vi "Dashboard Main.vi"() -> ()   [LabVIEW 2020]
uses:
  <vilib>/event_ctls.llb/eventvkey.ctl
  <vilib>/Rock Robotics/Network Tables/NT Read Numeric Array.vi
  <vilib>/Rock Robotics/WPI/Dashboard/WPI_DashboardLogging Global.vi
panel:
  in  "Camera Settings Right":T1={"Frame Rate"=30, "Compression"=30, "Size"=1, "DB Camera Config"=FALSE} {"Frame Rate" scale=1.0..30.0; "Compression" scale=100.0..-1.0; "Size" items=["640x480", "320x240", "160x120"]}
  in  "Camera Name Right":string(combo)="No Camera Selection"
  out "Camera Perf":string
  in  "Camera Settings":T1={"Frame Rate"=30, "Compression"=30, "Size"=1, "DB Camera Config"=FALSE} {"Frame Rate" scale=1.0..30.0; "Compression" scale=100.0..-1.0; "Size" items=["640x480", "320x240", "160x120"]}
  in  "TCP":refnum<k5>
  in  "Rec Mode":enum32{"Stop", "Record", "Playback"}(radio)
  out "Robot IP":string
  out "Image Message":string="Timeout in Camera Communications"
  in  "Dashboard Tab":T2(tab)
  in  "Select Auto":string(combo)="Select Autonomous ..."
  out "NT Connection":bool
  out "MotorChart R":cluster{"Numeric":dbl, "Numeric":dbl}(graph)
  out "MotorChart L":cluster{"Numeric":dbl, "Numeric":dbl}(graph)
  out "MotorSliders R":cluster{"MotorSlide1":dbl, "MotorSlide2":dbl} {"MotorSlide2" scale=-1.0..1.0 scale format="%#_2e"; "MotorSlide1" scale=-1.0..1.0 scale format="%#_2e"}
  out "MotorSliders L":cluster{"MotorSlide1":dbl, "MotorSlide2":dbl} {"MotorSlide2" scale=-1.0..1.0 scale format="%#_2e"; "MotorSlide1" scale=-1.0..1.0 scale format="%#_2e"}
  out "Gyro":dbl(knob) scale=0.0..360.0
  out "JS1 Z":dbl(slide) scale=-1.0..1.0 scale format="%#_2e"
  out "JS1 Graph":cluster{"X":dbl, "Y":dbl}[](graph)
  out "JS1 Buttons":T3
  out "JS2 Z":dbl(slide) scale=-1.0..1.0 scale format="%#_2e"
  out "JS2 Graph":cluster{"X":dbl, "Y":dbl}[](graph)
  out "JS2 Buttons":T3
  out "Mode":T4(ring)=enum."Auto Disabled"
  out "Right Camera Perf":cluster{"Bandwidth (Mbps)":dbl, "FPS":dbl}
  out "Camera Image Right":T5(plugin-control)
  in  "DB/String 9":string
  in  "DB/String 8":string
  in  "DB/String 7":string
  in  "DB/String 6":string
  in  "DB/String 5":string
  in  "DB/String 4":string
  in  "DB/String 3":string
  in  "DB/String 2":string
  in  "DB/String 1":string
  in  "DB/String 0":string
  in  "DB/Slider 0":dbl(slide) scale=0.0..5.0
  in  "DB/Slider 1":dbl(slide) scale=0.0..5.0
  in  "DB/Slider 2":dbl(slide) scale=0.0..5.0
  in  "DB/Slider 3":dbl(slide) scale=0.0..5.0
  out "DB/LED 3":bool
  out "DB/LED 2":bool
  out "DB/LED 1":bool
  out "DB/LED 0":bool
  in  "DB/Button 3":bool
  in  "DB/Button 2":bool
  in  "DB/Button 1":bool
  in  "DB/Button 0":bool caption="New Name"
  out "armMaximumPosition":dbl
  out "armMinimumPosition":dbl
  out "armCmdSetpoint":dbl
  out "armSetpoint":dbl
  out "armSensor Position":dbl
  out "navX Heading":dbl
  out "navX Pitch":dbl
  out "navX Roll":dbl
  out "navX Yaw":dbl
  in  "select Teleop":i32=1
  in  "Test Slider":dbl(slide) scale=0.0..100.0 scale format="%#_3g"
  in  "On/Off":bool caption="Solenoid"
  in  "Test Name":u16(ring) items=["Select the test to run..."]
  in  "Test Tree":string(tree)
  in  "Motor":cluster{"Value":dbl, "Enable":bool} {"Value" scale=-1.0..1.0 scale format="%#_3g"}
  out "Progress":T6 {"Test Progress" scale=0.0..100.0}
  in  "Rev/Fwd":cluster{"Forward":bool, "Reverse":bool}
  in  "Test Ring":u16(ring) items=["Monochrome", "Color"]
  in  "CheckList":i32(listbox)
  out "Tree":string(tree)
  out "Camera Image":T5(plugin-control)
  out "Background":bool
  in  "Camera Name":string(combo)="No Camera Selection"
  # "HW"
  # "HW"
  # "Joysticks"
  # "Drive Motors"
  # "Front"
  # "Right"
  # "Left"
  # "Back"
  # "This tab is a great place for autonomous settings and robot-specific values.\nPlace controls and indicators inside this tab and match name to\nDashboard Variables on robot. You can also delete this comment."
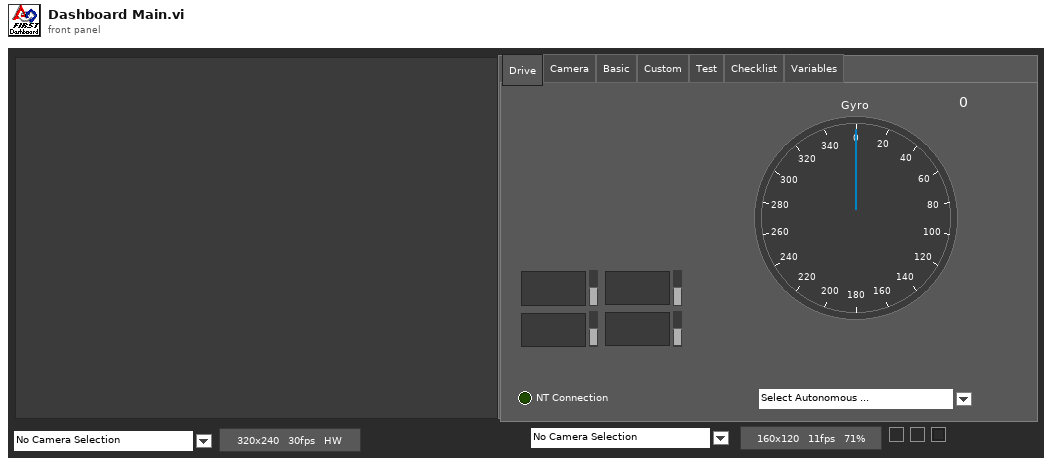
[diagram p1: front panel]
types:
  T1 = cluster{"Frame Rate":i32, "Compression":i32, "Size":u16, "DB Camera Config":bool}
  T2 = enum32{"Drive", "Camera", "Basic", "Custom", "Test", "Checklist", "Variables"}
  T3 = cluster{bool, bool, bool, bool, bool, bool, bool, bool, bool, bool, bool, bool}
  T4 = enum8{"Tele-Op Disabled", "Tele-Op Enabled", "Auto Disabled", "Auto Enabled", "Test Disabled", "Test Enabled", "Disconnected", "No Code", "E-Stop"}
  T5 = typedef "IMAQ Image.ctl" = refnum<image>
  T6 = cluster{"Test Progress":u8, "Test Progress Text":string}
  T7 = cluster{"Save Path":path, "Interval (s)":dbl, "Keep":i32}
  T8 = enum32{"Drive", "Camera", "Basic", "Custom", "Test", "Commands", "Checklist", "Variables"}
  T9 = typedef "Image Type" = u32
  T10 = cluster{"Global Rectangle":i32[], "Contours":cluster{"Contour Type":u32, "ROI Type":u32, "Points":i32[]}[]}
  T11 = cluster{"Camera Name":string, string, "Saved DB Images Info":cluster{"Save Path":path, "Interval (s)":dbl, "Keep":i32}}
  T12 = cluster{"Camera Name Right":string, string, "Saved DB Images Info":cluster{"Save Path":path, "Interval (s)":dbl, "Keep":i32}}
  T13 = cluster{"Camera Image":refnum<vi>, "Dashboard Tab":refnum<vi>, "Background":refnum<vi>, "Rec Mode":refnum<vi>, "Test Slider":refnum<vi>, "On/Off ":refnum<vi>, "Test Ring":refnum<vi>, "Rev/Fwd":refnum<vi>, "Test Name":refnum<vi>, "Motor":refnum<vi>, "Progress":refnum<vi>, "CheckList":refnum<vi>, "Tree":refnum<vi>, "Test Tree":refnum<vi>, "Camera Settings":refnum<vi>, "Camera Name":refnum<vi>, "Camera Perf":refnum<vi>, "Camera Settings Right":refnum<vi>, "Camera Name Right":refnum<vi>, "Camera Image Right":refnum<vi>}
  T14 = cluster{"Error Strings":string, "Disable Counts":cluster{u16, u16}, "Rail Faults":cluster{u16, u16, u16}, "Robot IP":string, "DB Mode":u8, "Event Info":cluster{"Name":string, "Type":u8, "Number":u16, "Replay":u8}}
  T15 = cluster{"Storage":cluster{"Disk Free":u64, "RAM Block":u32, "RAM free":u32}, "CPU Utilization":cluster{"CPU % ISR":sgl, "CPU % Time Crit":sgl, "CPU % Timed Str":sgl, "CPU % High":sgl, "CPU % Above":sgl, "CPU % Normal":sgl, "CPU % Low":sgl}, "CAN":cluster{"% Bus Utilization":sgl, "Bus Off Cnt":u32, "TX_FIFO Full Cnt":u32, "Receive Error Cnt":u8, "Transmit Error Cnt":u8}, "HID":cluster{"HID Outputs":u32, "Rumble Low":u16, "Rumble High":u16}[]}
  T16 = cluster{"Status bits":cluster{"Test Mode":bool, "Autonomous":bool, "Enabled":bool, "Code Start":bool, "Brownout":bool, "Reserved 2":bool, "Reserved 3":bool, "E-Stop":bool}, "Code Trace":cluster{"Disabled":bool, "TeleOp":bool, "Auto":bool, "Test":bool}, "Controller Type":enum16{"unknown", "cRIO", "roboRio"}, "Code?":enum16{"unknown", "noCode", "code"}, "Battery V":dbl}
  T17 = cluster{"Control Bits":cluster{"TestMode":bool, "Autonomous":bool, "Enabled":bool, "FMS Present":bool, bool, bool, bool, "E-Stop":bool}, "Team Station ":u8, "Countdown":sgl, "Joystick Values":cluster{"Axes":dbl[], "Buttons":bool[], "POVs":i16[]}[]}
  T18 = cluster{"Axes":dbl[], "Buttons":bool[], "POVs":i16[]}[]
  T19 = cluster{"Axes":dbl[], "Buttons":bool[], "POVs":i16[]}
  T20 = cluster{"Buttons[0]":bool, "Buttons[1]":bool, "Buttons[2]":bool, "Buttons[3]":bool, "Buttons[4]":bool, "Buttons[5]":bool, "Buttons[6]":bool, "Buttons[7]":bool, "Buttons[8]":bool, "Buttons[9]":bool, "Buttons[10]":bool, "Buttons[11]":bool}
  T21 = cluster{"Operation":enum16{"Update", "Clear"}, "Color Box":u32}[]
  T22 = typedef "eventvkey.ctl" = enum16{"ASCII", "Enter", "Return", "Shift", "Ctrl", "Alt", "Cmd", "Opt", "Caps", "NumLock", "Clear", "Break", "Up", "Down", "Left", "Right", "Insert", "Delete", "Home", "End", "PageUp", "PageDown", "Escape", "Help", "Pause", "ScrollLock", "F1", "F2", "F3", "F4", "F5", "F6", "F7", "F8", "F9", "F10", "F11", "F12", "F13", "F14", "F15", "F16", "F17", "F18", "F19", "F20", "F21", "F22", "F23", "F24", "Play", "VolumeUp", "VolumeDown", "Mute", "Two Byte Char"}
  T23 = cluster{"Image Size":bool, "Image Type":bool, "Pixel Value":bool, "ROI Information":bool, "Zoom Factor":bool}
  T24 = cluster{"Operation":enum16{"Update", "Clear"}, "Color Box":u32}
  T25 = cluster{"Shift":bool, "Ctrl":bool, "Alt":bool, "Cmd":bool, "Opt":bool}
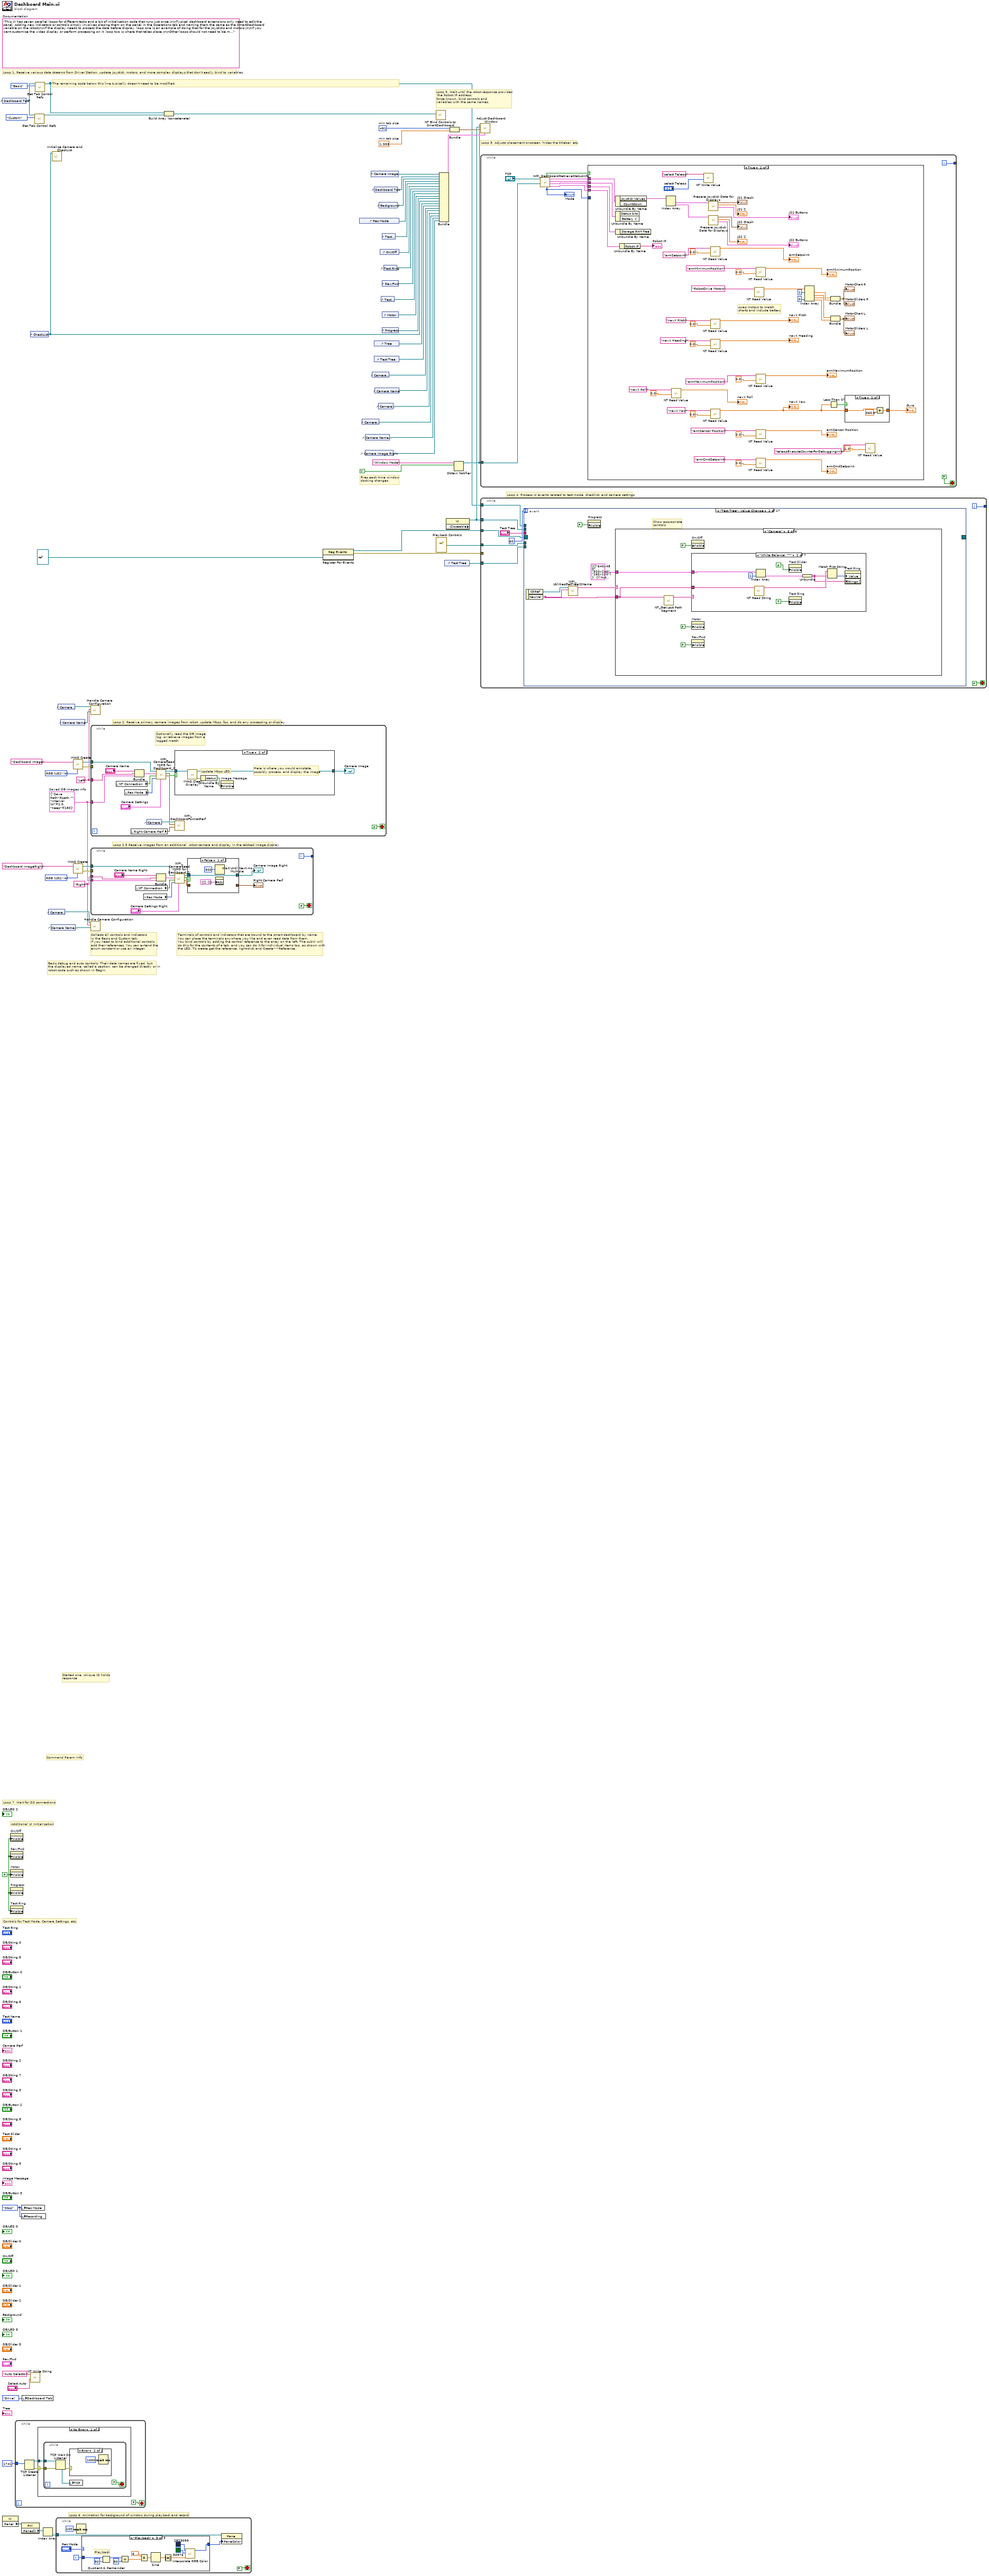
[diagram p0: block diagram]
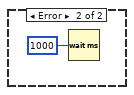
[diagram p4: hidden frame]
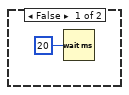
[diagram p5: hidden frame]
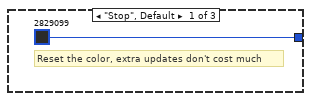
[diagram p7: hidden frame]
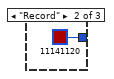
[diagram p8: hidden frame]
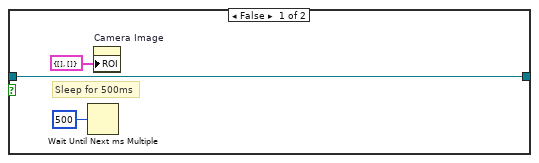
[diagram p9: hidden frame]
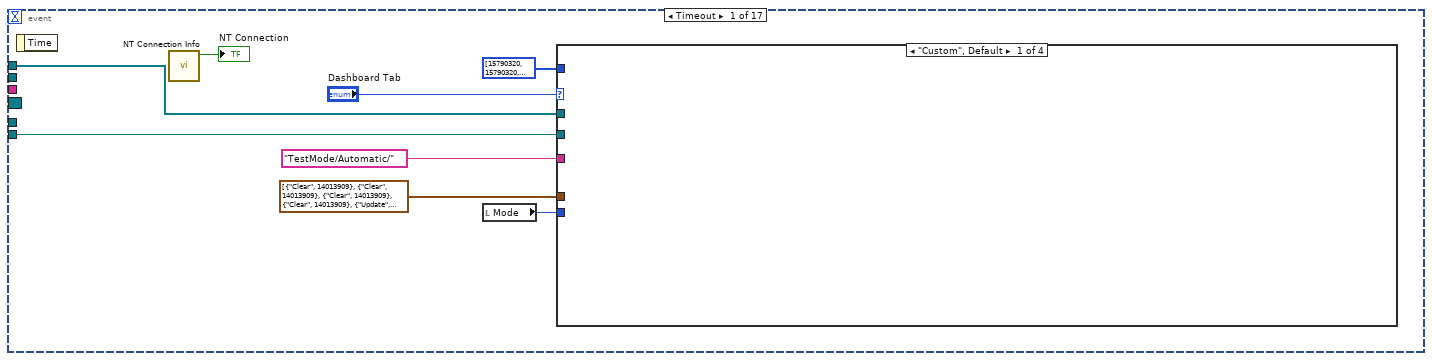
[diagram p10: hidden frame]
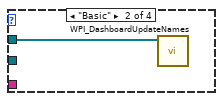
[diagram p11: hidden frame]
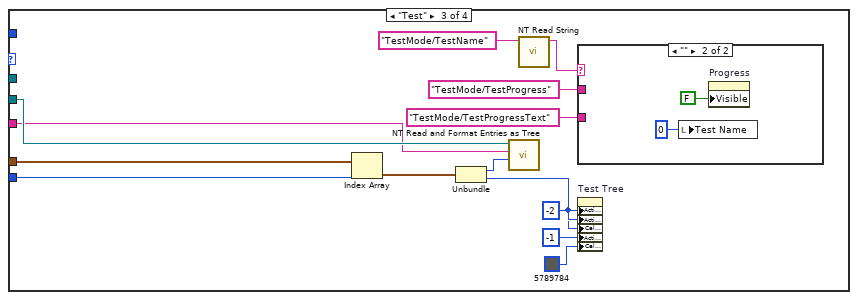
[diagram p12: hidden frame]
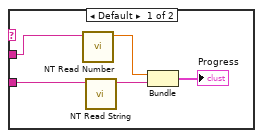
[diagram p13: hidden frame]
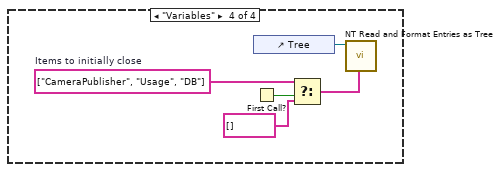
[diagram p14: hidden frame]
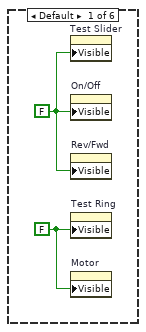
[diagram p15: hidden frame]
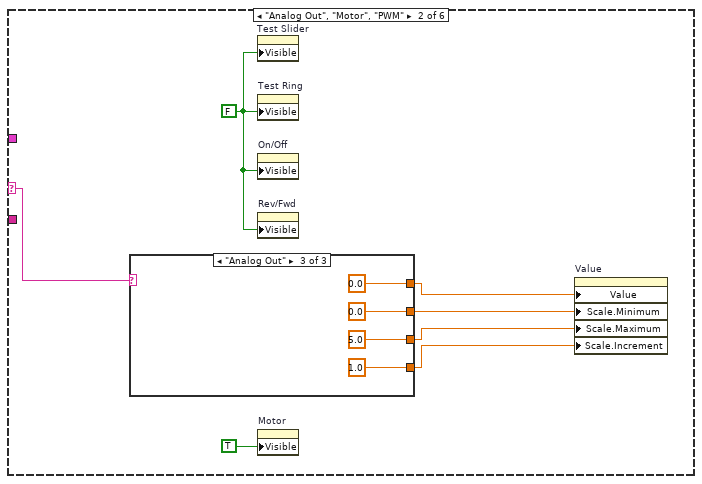
[diagram p16: hidden frame]
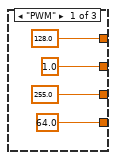
[diagram p17: hidden frame]
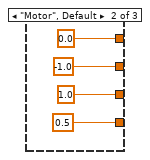
[diagram p18: hidden frame]
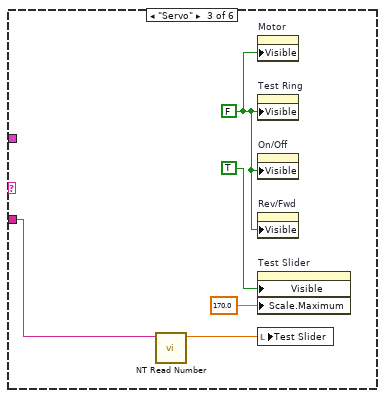
[diagram p19: hidden frame]
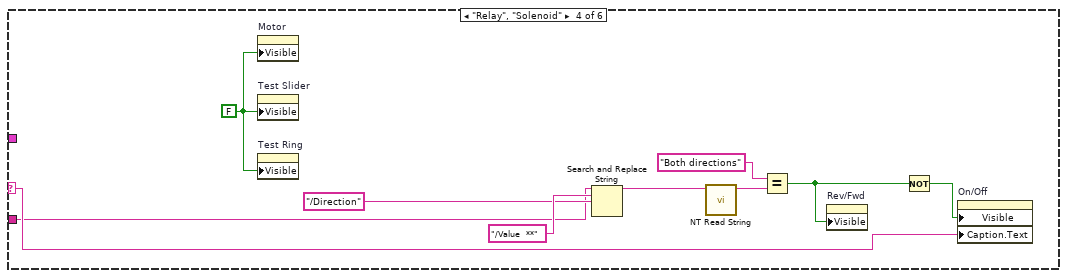
[diagram p20: hidden frame]
diagram:
  w3 = T7 {"Save Path"=path "", "Interval (s)"=1.0, "Keep"=180}  # Saved DB Images Info
  w2 = "Right"
  w1 = "Left"
  w13 = T9 4 items=["Grayscale (U8)", "Grayscale (I16)", "Grayscale (SGL)", "Complex (CSG)", "RGB (U32)", "HSL (U32)", "RGB (U64)"] ("Image Type")
  w42 = 491  # min tab size
  w41 = 1.333  # min tab size
  w49 = enum32{"Stop", "Record", "Playback"}."Stop" ("Rec Mode")
  w26 = FALSE ("Visible")
  (unwired) "This VI has seven parallel loops for different tasks and a bit of initialization code that runs just once.\n\nTypical dashboard extensions only need to edit the panel. Adding new indicators or controls simply involves placing them on the panel in the Operations tab and naming them the same as the SmartDashboard variable on the robot\n\nIf the display needs to process the data before display, loop one is an example of doing that for the joysticks and motors.\n\nIf you want customize the video display or perform processing on it, loop two is where that takes place.\n\nOther loops should not need to be modified. They are pretty standard, and document the task they perform."  # Documentation
  w63 = T9 4 items=["Grayscale (U8)", "Grayscale (I16)", "Grayscale (SGL)", "Complex (CSG)", "RGB (U32)", "HSL (U32)", "RGB (U64)"] ("Image Type")
  # "Loop 2.5 Receive images from an additional  robot camera and display in the tabbed image display"
  # "Command Param Info"
  # "Started one, Unique ID holds\nresponse"
  # "Loop 7. Wait for DS connections"
  # "Basic debug and auto controls: Their data names are fixed, but\nthe displayed name, called a caption, can be changed directly or in\nrobot code such as shown in Begin."
  # "Controls for Test Mode, Camera Settings, etc."
  # "Additional UI Initialization"
  # "Loop 6. Animation for background of window during playback and record"
  # "Fires each time window\ndocking changes."
  # "Collects all controls and indicators\nin the Basic and Custom tab.\nIf you need to bind additional controls,\nadd their references. You can extend the\nenum constant or use an integer."
  # "The remaining code below this line typically doesn't need to be modified."
  # "Loop 4. Process UI events related to test mode, checklist, and camera settings"
  # "Terminals of controls and indicators that are bound to the smart dashboard by name.\nYou can place the terminals anywhere you like and even read data from them.\nYou bind controls by adding the control reference to the array on the left. The subVI will\ndo this for the contents of a tab, and you can do it for individual items too, as shown with\nthe LED. To create get the reference, right-click and Create>>Reference."
  # "Loop 3. Wait until the robot response provides\n the Robot IP address.\nOnce known, bind controls and\nvariables with the same names."
  # "Loop 5. Adjusts placement onscreen, hides the titlebar, etc."
  # "Loop 1. Receive various data streams from Driver Station, update joystick, motors, and more complex displays that don't easily bind to variables."
  # "Loop 2. Receive primary camera images from robot, update Mbps, fps, and do any processing or display"
  n1 = control-ref of="Dashboard Tab"() -> (w47:refnum<vi>)
  n2 = property class="VI"() -> ("Panel"=w55:refnum<vi>)  [unwired: 2 in, 2 out]
  n3 = property on="On/Off" class="Bool (strict)"("Visible"=w26) -> ()  [unwired: 2 in, 2 out]
  n4 = property on="Rev/Fwd" class="Clust (strict)"("Visible"=w26) -> ()  [unwired: 2 in, 2 out]
  n5 = property on="Motor" class="Clust (strict)"("Visible"=w26) -> ()  [unwired: 2 in, 2 out]
  n6 = property on="Progress" class="Clust (strict)"("Visible"=w26) -> ()  [unwired: 2 in, 2 out]
  n7 = property on="Test Ring" class="Ring (strict)"("Visible"=w26) -> ()  [unwired: 2 in, 2 out]
  n8 = while {
    tunnel: u16 1741 ("timeout ms (25000)") -> [w65]
    stop <- FALSE stop-if-true
    n9 = TCP Create Listener(10:w65) -> (0:w64:errorcluster, 3:w66:refnum<k5>)  [unwired: 4 in, 1 out]
    n10 = case shown="No Error" w64 {
      selector: w64 -> [w68 _]
      tunnel: w66 -> [w69 _]
      frame No Error {
        n11 = while {
          tunnel: w69 -> [w72]
          tunnel: w68 -> [w71]
          stop <- FALSE stop-if-true
          n12 = TCP Wait On Listener(8:w71, 11:w72) -> (0:w73:errorcluster, 4:w74:refnum<k5>)  [unwired: 2 in, 3 out]
          n13 = case shown="Error" w73 {
            frame No Error {
            }
            frame Error {
              n14 = Wait (ms)(milliseconds to wait=u32 1000) -> ()  [unwired: 1 out]
            }
          }
          n15 = local write "TCP"(w74) -> ()
        }
      }
      frame Error {
        n16 = Wait (ms)(milliseconds to wait=u32 1000) -> ()  [unwired: 1 out]
      }
    }
  }
  n17 = local write "Rec Mode"(w49) -> ()
  n18 = global write "WPI_DashboardLogging Global.vi" "Recording"(w49) -> ()
  n19 = property class="Pnl"(reference=w55) -> ("Panes[]"=w56:refnum<vi>[])  [unwired: 1 in, 2 out]
  n20 = local write "Dashboard Tab"(T2."Drive" ("Dashboard Tab")) -> ()
  n21 = call <vilib>:"NT Write String.vi"("value"="Select Auto", "name"="Auto Selector" ("Name")) -> ()  [unwired: 9 in, 1 out]
  n22 = control-ref of="CheckList"() -> (w37:refnum<vi>)
  n23 = call <vilib>:"Get Tab Control Refs.vi"("Page Index"=T8."Custom" ("Dashboard Tab"), "TabControl in"=w47) -> ("ControlsOnPage"=w46:refnum<vi>[])  [unwired: 9 in]
  n24 = call <vilib>:"Get Tab Control Refs.vi"("Page Index"=T8."Basic" ("Dashboard Tab"), "TabControl in"=w47) -> ("ControlsOnPage"=w17:refnum<vi>[])  [unwired: 9 in]
  n25 = Index Array(array=w56) -> (element=w54:refnum<vi>)  [unwired: 1 in]
  n26 = control-ref of="Camera Settings Right"() -> (w10:refnum<vi>)
  n27 = control-ref of="Camera Name Right"() -> (w9:refnum<vi>)
  n28 = call "Initialize Camera and CheckList.vi"("ListBox in"=w37) -> ()  [unwired: 11 in]
  n29 = while {
    tunnel: w54 -> [w78]
    i -> [w81]
    stop <- FALSE stop-if-true
    n30 = Wait (ms)(milliseconds to wait=u32 100) -> ()  [unwired: 1 out]
    n31 = case shown="\"Playback\"" "Rec Mode" {
      tunnel: w81 -> [_ _ w96]
      tunnel: [u32 2829099 ("Base Color") u32 11141120 ("Target Color") w85] -> w77
      frame "Stop", Default {
        # "Reset the color, extra updates don't cost much"
      }
      frame "Record" {
      }
      frame "Playback" {
        # "Playback"
        n32 = Quotient & Remainder(x=w96, y=u32 50 ("milliseconds to wait")) -> (x-y*floor(x/y)=w92:u32)  [unwired: 1 out]
        n33 = Divide(x=w92, y=u32 50 ("milliseconds to wait")) -> (x/y=w89:dbl)
        n34 = Multiply(x=6.283185307179586, y=w89) -> (x*y=w94:dbl)
        n35 = Sine(x=w94) -> (sin(x)=w93:dbl)
        n36 = Absolute Value(x=w93) -> (abs(x)=w86:dbl)
        n37 = call "Interpolate RGB Color.vi"("Proportion"=w86, "Target Color"=u32 30976, "Base Color"=u32 2829099) -> ("Result Color"=w85:u32)  [unwired: 8 in]
      }
    }
    n38 = property class="Pane"(reference=w78, "PaneColor"=w77) -> ()  [unwired: 1 in, 2 out]
  }
  n39 = control-ref of="Camera Settings"() -> (w22:refnum<vi>)
  n40 = control-ref of="Camera Name"() -> (w21:refnum<vi>)
  n41 = call "IMAQ Create"("Image Name"="Dashboard Image", "Image Type"=w63) -> ("New Image"=w61:T5, "error out"=w60:errorcluster)  [unwired: 2 in, 1 out]
  n42 = call "IMAQ Create"("Image Name"="Dashboard ImageRight", "Image Type"=w13) -> ("New Image"=w12:T5, "error out"=w11:errorcluster)  [unwired: 2 in, 1 out]
  n43 = call "Handle Camera Configuration.vi"("CameraNameRef"=w21, "Display Name"=w1, "ClusterRef"=w22) -> ()  [unwired: 9 in]
  n44 = while {
    tunnel: w61 -> [w110]
    tunnel: w60 -> [_]
    tunnel: w3 -> [w103]
    tunnel: w1 -> [w100]
    stop <- FALSE stop-if-true
    # "Optionally read the DB image,\nlog, or retrieve images from a\nlogged match"
    n45 = local read "NT Connection"() -> (w104:bool)
    n46 = local read "Rec Mode"() -> (w107:enum32{"Stop", "Record", "Playback"})
    n47 = local read "Right Camera Perf"() -> (w98:cluster{"Bandwidth (Mbps)":dbl, "FPS":dbl})
    n48 = Bundle("Camera Name"="Camera Name", w100, "Saved DB Images Info"=w103) -> (w102:T11)  [unwired: 1 in]
    n49 = control-ref of="Camera Perf"() -> (w97:refnum<vi>)
    n50 = call <vilib>:"WPI_CameraRead MJPG for Dashboard_2.vi"("Camera Settings"="Camera Settings", "Rec Mode"=w107, "NT Connection"=w104, "Capture Info"=w102, "Image in"=w110) -> ("perf info"=w99:cluster{"Bandwidth (Mbps)":dbl, "fps":dbl}, "Active"=w108:bool, "Image\\ out"=w109:T5)  [unwired: 4 in]
    n51 = case shown="True" w108 {
      tunnel: w109 -> [w113 w116]
      tunnel: [w113 w115] -> w105
      frame False {
        # "Sleep for 500ms"
        n52 = Wait Until Next ms Multiple(millisecond multiple=u32 500) -> ()  [unwired: 1 out]
        n53 = property on="Camera Image" class="ImageControl"("ROI"=T10 {"Global Rectangle"=[], "Contours"=[]}) -> ()  [unwired: 2 in, 2 out]
      }
      frame True {
        # "Here is where you would annotate,\npossibly process, and display the image"
        # "Update Mbps LED"
        n54 = call "IMAQ Clear Overlay"("Image"=w116) -> ("error out"=w117:errorcluster, "Image Out"=w115:T5)  [unwired: 2 in, 7 out]
        n55 = Unbundle By Name(w117) -> ("status"=w118:bool)
        n56 = property on="Image Message" class="Str"("Visible"=w118) -> ()  [unwired: 2 in, 2 out]
      }
    }
    "Camera Image" <- w105
    n57 = call <vilib>:"WPI_DashboardFormatPerf.vi"("Right Camera Perf"=w98, "Performance"=w99, "String in"=w97) -> ()  [unwired: 9 in]
  }
  n58 = while {
    tunnel: w12 -> [w133]
    tunnel: w11 -> [_]
    tunnel: [w128] -> _
    tunnel: w3 -> [w124]
    tunnel: w2 -> [w121]
    i -> [w128]
    stop <- FALSE stop-if-true
    n59 = local read "NT Connection"() -> (w125:bool)
    n60 = local read "Rec Mode"() -> (w132:enum32{"Stop", "Record", "Playback"})
    n61 = Bundle("Camera Name Right"="Camera Name Right", w121, "Saved DB Images Info"=w124) -> (w123:T12)  [unwired: 1 in]
    n62 = call <vilib>:"WPI_CameraRead MJPG for Dashboard_2.vi"("Camera Settings"="Camera Settings Right", "Rec Mode"=w132, "NT Connection"=w125, "Capture Info"=w123, "Image in"=w133) -> ("perf info"=w119:cluster{"Bandwidth (Mbps)":dbl, "fps":dbl}, "Active"=w127:bool, "Image\\ out"=w130:T5)  [unwired: 4 in]
    n63 = case shown="False" w127 {
      tunnel: w130 -> [w135 w138]
      tunnel: [w135 w138] -> w126
      tunnel: [_ w137] -> w120
      tunnel: w119 -> [_ w137]
      frame False {
        n64 = Wait Until Next ms Multiple(millisecond multiple=u32 500) -> ()  [unwired: 1 out]
        n65 = property on="Camera Image Right" class="ImageControl"("ROI"=T10 {"Global Rectangle"=[], "Contours"=[]}) -> ()  [unwired: 2 in, 2 out]
      }
      frame True {
      }
    }
    "Camera Image Right" <- w126
    "Right Camera Perf" <- w120
  }
  n66 = call "Handle Camera Configuration.vi"("CameraNameRef"=w9, "Display Name"=w2, "ClusterRef"=w10) -> ()  [unwired: 9 in]
  n67 = Build Array (concatenate)(w17, w46) -> (w45:refnum<vi>[])
  n68 = register-events(refnum<vi> refnum) -> (reference out=w52:refnum<event-registration>, error out=w51:errorcluster)  [unwired: 2 in]
  n69 = control-ref of="Rec Mode"() -> (w32:refnum<vi>)
  n70 = control-ref of="Camera Settings Right"() -> (w8:refnum<vi>)
  n71 = control-ref of="Camera Name Right"() -> (w7:refnum<vi>)
  n72 = control-ref of="Camera Image Right"() -> (w6:refnum<vi>)
  n73 = control-ref of="Camera Image"() -> (w44:refnum<vi>)
  n74 = control-ref of="Camera Settings"() -> (w20:refnum<vi>)
  n75 = control-ref of="Dashboard Tab"() -> (w43:refnum<vi>)
  n76 = control-ref of="Tree"() -> (w36:refnum<vi>)
  n77 = control-ref of="Test Tree"() -> (w35:refnum<vi>)
  n78 = control-ref of="Camera Name"() -> (w19:refnum<vi>)
  n79 = control-ref of="Camera Perf"() -> (w18:refnum<vi>)
  n80 = control-ref of="Background"() -> (w39:refnum<vi>)
  n81 = control-ref of="On/Off"() -> (w30:refnum<vi>)
  n82 = control-ref of="Test Name"() -> (w34:refnum<vi>)
  n83 = control-ref of="Test Slider"() -> (w31:refnum<vi>)
  n84 = control-ref of="Rev/Fwd"() -> (w28:refnum<vi>)
  n85 = control-ref of="Motor"() -> (w33:refnum<vi>)
  n86 = control-ref of="Progress"() -> (w27:refnum<vi>)
  n87 = control-ref of="Test Ring"() -> (w29:refnum<vi>)
  n88 = call <vilib>:"NT Bind Controls to SmartDashboard.vi"("Bound Control Refs"=w45) -> ()  [unwired: 11 in]
  n89 = vi-ref "Playback Controls.vi"() -> (w53:refnum<vi>)
  n90 = Bundle("Camera Image"=w44, "Dashboard Tab"=w43, "Background"=w39, "Rec Mode"=w32, "Test Slider"=w31, "On/Off"=w30, "Test Ring"=w29, "Rev/Fwd"=w28, "Test Name"=w34, "Motor"=w33, "Progress"=w27, "CheckList"=w37, "Tree"=w36, "Test Tree"=w35, "Camera Settings"=w20, "Camera Name"=w19, "Camera Perf"=w18, "Camera Settings Right"=w8, "Camera Name Right"=w7, "Camera Image Right"=w6) -> (w38:T13)  [unwired: 1 in]
  n91 = control-ref of="Test Tree"() -> (w57:refnum<vi>)
  n92 = property class="VI" props=["Front Panel.Closeable"]() -> (reference out=w48:refnum<vi>)  [unwired: 2 in, 2 out]
  n93 = Bundle("min tab size"=w42, "min tab size"=w41) -> (w40:cluster{"min tab size":i32, "min tab size":dbl})  [unwired: 1 in]
  n94 = Obtain Notifier(name (unnamed)="Window Mode", notification data type=TRUE) -> (notifier out=w25:refnum<notifier>)  [unwired: 2 in, 2 out]
  n95 = call "Adjust Dashboard Window.vi"("Sizing Refnums"=w38, "Size Constraints"=w40, "VI"=w48, "WIn Mode"=w25) -> ()  [unwired: 8 in]
  n96 = while {
    tunnel: [w147] -> _
    tunnel: w25 -> [w139]
    i -> [w147]
    stop <- FALSE stop-if-true
    n97 = call <vilib>:"WPI_DashboardRetrieveStatusInfo.vi"("Window Mode Notifier"=w139, "TCP Cnx"="TCP") -> ("Power and Errors"=w142:T14, "Robot Metrics"=w145:T15, "Status Info"=w146:T16, "Control Info"=w143:T17, "Robot Mode"=w141:T4, "Process?"=w144:bool)  [unwired: 4 in]
    "Mode" <- w141
    n98 = case shown="True" w144 {
      tunnel: w146 -> [_ w206]
      tunnel: w145 -> [_ w205]
      tunnel: w143 -> [_ w204]
      tunnel: w142 -> [_ w203]
      tunnel: w141 -> [_ _]
      frame False {
        n99 = Wait (ms)(milliseconds to wait=u32 20) -> ()  [unwired: 1 out]
      }
      frame True {
        # "swap motors to match\ncharts and include battery"
        n100 = Unbundle By Name(w204) -> ("Joystick Values"=w194:T18)  [unwired: 1 out]
        n101 = Unbundle By Name(w206) -> ()  [unwired: 2 out]
        n102 = Unbundle By Name(w205) -> ()  [unwired: 1 out]
        n103 = Unbundle By Name(w203) -> ("Robot IP"=→"Robot IP":string)
        n104 = Index Array(array=w194) -> (element #1=w193:T19, element #2=w189:T19)  [unwired: 2 in]
        n105 = call-poly <vilib>:"NT Read Value.vi"("default value"=0.0, "name"="navX Roll") -> ("value"=→"navX Roll":dbl)  [unwired: 7 in, 2 out]
        n106 = call-poly <vilib>:"NT Write Value.vi"("value"="select Teleop", "name"="select Teleop") -> ()  [unwired: 9 in, 1 out]
        n107 = call "Prepare Joystick Data for Displays.vi"("Joystick Values"=w193) -> ("Buttons"=→"JS1 Buttons":T20, "Z Axis"=→"JS1 Z":dbl, "Cartesian Data"=→"JS1 Graph":cluster{"X axis":dbl, "X axis":dbl}[])  [unwired: 8 in]
        n108 = call "Prepare Joystick Data for Displays.vi"("Joystick Values"=w189) -> ("Buttons"=→"JS2 Buttons":T20, "Z Axis"=→"JS2 Z":dbl, "Cartesian Data"=→"JS2 Graph":cluster{"X axis":dbl, "X axis":dbl}[])  [unwired: 8 in]
        n109 = call-poly <vilib>:"NT Read Value.vi"("default value"=0.0, "name"="armSetpoint") -> ("value"=→"armSetpoint":dbl)  [unwired: 7 in, 2 out]
        n110 = call-poly <vilib>:"NT Read Value.vi"("default value"=0.0, "name"="navX Pitch") -> ("value"=→"navX Pitch":dbl)  [unwired: 7 in, 2 out]
        n111 = call-poly <vilib>:"NT Read Value.vi"("default value"=0.0, "name"="navX Heading") -> ("value"=→"navX Heading":dbl)  [unwired: 7 in, 2 out]
        n112 = call-poly <vilib>:"NT Read Value.vi"("default value"=0.0, "name"="navX Yaw") -> ("value"=w176:dbl)  [unwired: 7 in, 2 out]
        "navX Yaw" <- w176
        n113 = call-poly <vilib>:"NT Read Value.vi"("name"="RobotDrive Motors" ("Name")) -> ("value"=w184:dbl[])  [unwired: 8 in, 2 out]
        n114 = call-poly <vilib>:"NT Read Value.vi"("default value"=0.0, "name"="armMinimumPosition") -> ("value"=→"armMinimumPosition":dbl)  [unwired: 7 in, 2 out]
        n115 = call-poly <vilib>:"NT Read Value.vi"("default value"=0.0, "name"="armMaximumPosition") -> ("value"=→"armMaximumPosition":dbl)  [unwired: 7 in, 2 out]
        n116 = call-poly <vilib>:"NT Read Value.vi"("default value"=0.0, "name"="armSensor Position") -> ("value"=→"armSensor Position":dbl)  [unwired: 7 in, 2 out]
        n117 = call-poly <vilib>:"NT Read Value.vi"("default value"=0.0, "name"="armCmdSetpoint") -> ("value"=→"armCmdSetpoint":dbl)  [unwired: 7 in, 2 out]
        n118 = Index Array(array=w184, index #1=1, index #4=0) -> (element #1=w198:dbl, element #2=w199:dbl, element #3=w197:dbl, element #4=w202:dbl)  [unwired: 2 in]
        n119 = Less Than 0?(x=w176) -> (x < 0?=w180:bool)
        n120 = Bundle("Numeric"=w197, "Numeric"=w198) -> (→"MotorChart R" →"MotorSliders R":cluster{"Numeric":dbl, "Numeric":dbl})  [unwired: 1 in]
        n121 = Bundle("Numeric"=w199, "Numeric"=w202) -> (→"MotorChart L" →"MotorSliders L":cluster{"Numeric":dbl, "Numeric":dbl})  [unwired: 1 in]
        n122 = case shown="True" w180 {
          tunnel: w176 -> [w207 w210]
          tunnel: [w207 w208] -> w179
          frame False {
          }
          frame True {
            n123 = Add(x=w210, y=360.0) -> (x+y=w208:dbl)
          }
        }
        "Gyro" <- w179
        n124 = call-poly <vilib>:"NT Read Value.vi"("default value"=-1.0, "name"="teleopExecuteCounterForDebuggingInit") -> ()  [unwired: 7 in, 3 out]
      }
    }
  }
  n125 = while {
    tunnel: [w216] -> _
    tunnel: w57 -> [w215]
    tunnel: w53 -> [w214]
    tunnel: w52 -> [w213]
    tunnel: w51 -> [_]
    tunnel: w48 -> [w212]
    tunnel: w17 -> [w211]
    i -> [w216]
    stop <- FALSE stop-if-true
    n126 = event shown="[1] \"Test Tree\": Value Change" {
      selector: w213 -> [_ _ _ _ _ _ _ _ _ _ _ _ _ _ _ _ _]
      dyn-events: [_ _ _ _ _ _ _ _ _ _ _ _ _ w421 _ _ _] -> _
      timeout: u32 60 ("milliseconds to wait") -> [_ _ _ _ _ _ _ _ _ _ _ _ _ _ _ _ _]
      tunnel: w215 -> [w226 _ _ _ _ _ _ _ _ _ _ _ _ _ _ _ _]
      tunnel: "Test Tree" -> [_ _ _ _ _ _ _ _ w394 w401 w402 w405 w412 _ _ _ _]
      tunnel: w214 -> [_ _ _ _ _ _ _ _ _ _ _ _ _ w423 _ w438 _]
      tunnel: w212 -> [_ _ _ _ _ _ _ _ _ _ _ _ _ w419 _ _ _]
      tunnel: w211 -> [w221 _ _ _ _ _ _ _ _ _ _ _ _ _ _ _ _]
      event Timeout {
        n127 = event-data() -> ()  [unwired: 1 in, 1 out]
        n128 = call <vilib>:"NT Connection Info.vi"() -> ("Connected"=→"NT Connection":bool)  [unwired: 11 in]
        n129 = local read "Mode"() -> (w224:T4)
        n130 = case shown="\"Custom\", Default" "Dashboard Tab" {
          tunnel: w226 -> [_ _ w242 _]
          tunnel: "TestMode/Automatic/" ("Name Pattern") -> [_ _ w241 _]
          tunnel: T21 [{"Operation"=enum."Clear", "Color Box"=14013909}, {"Operation"=enum."Clear", "Color Box"=14013909}, {"Operation"=enum."Clear", "Color Box"=14013909}, {"Operation"=enum."Clear", "Color Box"=14013909}, {"Operation"=enum."Update", "Color Box"=14013909}, {"Operation"=enum."Update", "Color Box"=16777215}, {"Operation"=enum."Clear", "Color Box"=14013909}, {"Operation"=enum."Clear", "Color Box"=14013909}, {"Operation"=enum."Clear", "Color Box"=14013909}] -> [_ _ w234 _]
          tunnel: w224 -> [_ _ w233 _]
          tunnel: u32[] [15790320, 15790320, 15790320, 15790320, 16777215, 16777215, 15790320, 15790320, 15790320] -> [_ _ _ _]
          tunnel: w221 -> [_ w228 _ _]
          frame "Custom", Default {
          }
          frame "Basic" {
            n131 = call <vilib>:"WPI_DashboardUpdateNames.vi"("Controls on Tab"=w228) -> ()  [unwired: 11 in]
          }
          frame "Test" {
            w240 = -2 ("Active Item:Row Number")
            n132 = Index Array(array=w234, index=w233) -> (element=w235:T24)
            n133 = Unbundle(w235) -> ("Operation"=w236:enum16{"Update", "Clear"}, "Color Box"=w237:u32)
            n134 = call <vilib>:"NT Read and Format Entries as Tree.vi"("Operation"=w236, "Name Pattern"=w241, "Tree Refnum"=w242) -> ()  [unwired: 7 in, 2 out]
            n135 = call <vilib>:"NT Read String.vi"("name"="TestMode/TestName" ("Name")) -> ("value"=w231:string)  [unwired: 8 in, 2 out]
            n136 = case shown="\"\"" w231 {
              tunnel: "TestMode/TestProgress" ("Name") -> [w244 _]
              tunnel: "TestMode/TestProgressText" ("Name") -> [w243 _]
              frame Default {
                n137 = call <vilib>:"NT Read Number.vi"("name"=w244) -> ("value"=w245:dbl)  [unwired: 8 in, 2 out]
                n138 = call <vilib>:"NT Read String.vi"("name"=w243) -> ("value"=w246:string)  [unwired: 8 in, 2 out]
                n139 = Bundle("value"=w245, "value"=w246) -> (→"Progress":cluster{"value":dbl, "value":string})  [unwired: 1 in]
              }
              frame "" {
                n140 = local write "Test Name"(u16 0) -> ()
                n141 = property on="Progress" class="Clust (strict)"("Visible"=FALSE) -> ()  [unwired: 2 in, 2 out]
              }
            }
            n142 = property on="Test Tree" class="Tree (strict)"("Active Item Row Number"=w240, "ActiveColNum"=w240, "CellBG"=w237, "Active Item Row Number"=-1 ("Active Item:Row Number"), "CellBG"=u32 5789784 ("Color Box")) -> ()  [unwired: 2 in, 2 out]
          }
          frame "Variables" {
            w252 = string[] ["CameraPublisher", "Usage", "DB"]  # Items to initially close
            n143 = First Call?() -> (First Call?: T/F=w253:bool)
            n144 = control-ref of="Tree"() -> (w254:refnum<vi>)
            n145 = Select(t=w252, s=w253, f=string[] []) -> (s? t:f=w250:string[])
            n146 = call <vilib>:"NT Read and Format Entries as Tree.vi"("Tags to  Close"=w250, "Tree Refnum"=w254) -> ()  [unwired: 8 in, 2 out]
          }
        }
      }
      event "Test Tree": Value Change {
        # "Show appropriate\ncontrols"
        n147 = event-data() -> ("CtlRef"=w258:refnum<vi>, "NewVal"=w256:string)  [unwired: 1 in]
        n148 = call <vilib>:"WPI_UtilitiesGetTreeIOName.vi"("NewVal"=w256, "TreeControl in"=w258) -> ("I/O Name"=w259:string)  [unwired: 9 in]
        n149 = property on="Progress" class="Clust (strict)"("Visible"=FALSE) -> ()  [unwired: 2 in, 2 out]
        n150 = case shown="\"Camera\"" w259 {
          selector: w259 -> [_ w266 _ w288 w297 _]
          tunnel: w256 -> [_ _ w285 w287 _ w304]
          tunnel: cluster{string[]}[] [{["640x480", "320x240", "160x120"]}, {["Auto", "Fixed indoor", "Fixed outdoor 1", "Fixed outdoor 2", "Fixed fluorescent 1", "Fixed fluorescent 2", "Hold current"]}, {["Auto", "Flicker-free 50 Hz", "Flicker-free 60 Hz", "Hold current"]}, {["None", "Prioritize frame rate", "Prioritize image quality"]}, {["Monochrome", "Color"]}] -> [_ _ _ _ _ w303]
          frame Default {
            w261 = FALSE ("Visible")
            w260 = FALSE ("Visible")
            n151 = property on="Test Slider" class="Slide (strict)"("Visible"=w261) -> ()  [unwired: 2 in, 2 out]
            n152 = property on="On/Off" class="Bool (strict)"("Visible"=w261) -> ()  [unwired: 2 in, 2 out]
            n153 = property on="Rev/Fwd" class="Clust (strict)"("Visible"=w261) -> ()  [unwired: 2 in, 2 out]
            n154 = property on="Test Ring" class="Ring (strict)"("Visible"=w260) -> ()  [unwired: 2 in, 2 out]
            n155 = property on="Motor" class="Clust (strict)"("Visible"=w260) -> ()  [unwired: 2 in, 2 out]
          }
          frame "Analog Out", "Motor", "PWM" {
            w267 = FALSE ("Visible")
            n156 = case shown="\"Analog Out\"" w266 {
              tunnel: [1.0 ("Value") -1.0 ("Value") 0.0 ("Value")] -> w265
              tunnel: [255.0 ("Value") 1.0 ("Value") 5.0 ("Value")] -> w264
              tunnel: [128.0 ("Value") 0.0 ("Value") 0.0 ("Value")] -> w263
              tunnel: [64.0 ("Value") 0.5 ("Value") 1.0 ("Value")] -> w262
              frame "PWM" {
              }
              frame "Motor", Default {
              }
              frame "Analog Out" {
              }
            }
            n157 = property on="Test Slider" class="Slide (strict)"("Visible"=w267) -> ()  [unwired: 2 in, 2 out]
            n158 = property on="Test Ring" class="Ring (strict)"("Visible"=w267) -> ()  [unwired: 2 in, 2 out]
            n159 = property on="On/Off" class="Bool (strict)"("Visible"=w267) -> ()  [unwired: 2 in, 2 out]
            n160 = property on="Rev/Fwd" class="Clust (strict)"("Visible"=w267) -> ()  [unwired: 2 in, 2 out]
            n161 = property on="Motor" class="Clust (strict)"("Visible"=TRUE) -> ()  [unwired: 2 in, 2 out]
            n162 = property on="Value" class="Slide (strict)"("Value"=w263, "Scale.Minimum"=w265, "Scale.Maximum"=w264, "Scale.Increment"=w262) -> ()  [unwired: 2 in, 2 out]
          }
          frame "Servo" {
            w283 = FALSE ("Visible")
            n163 = call <vilib>:"NT Read Number.vi"("name"=w285) -> ("value"=w284:dbl)  [unwired: 8 in, 2 out]
            n164 = property on="Motor" class="Clust (strict)"("Visible"=w283) -> ()  [unwired: 2 in, 2 out]
            n165 = property on="Test Ring" class="Ring (strict)"("Visible"=w283) -> ()  [unwired: 2 in, 2 out]
            n166 = property on="On/Off" class="Bool (strict)"("Visible"=w283) -> ()  [unwired: 2 in, 2 out]
            n167 = property on="Rev/Fwd" class="Clust (strict)"("Visible"=w283) -> ()  [unwired: 2 in, 2 out]
            n168 = property on="Test Slider" class="Slide (strict)"("Visible"=TRUE, "Scale.Maximum"=170.0 ("Scale.Range:Maximum")) -> ()  [unwired: 2 in, 2 out]
            n169 = local write "Test Slider"(w284) -> ()
          }
          frame "Relay", "Solenoid" {
            w286 = FALSE ("Visible")
            n170 = property on="Motor" class="Clust (strict)"("Visible"=w286) -> ()  [unwired: 2 in, 2 out]
            n171 = property on="Test Slider" class="Slide (strict)"("Visible"=w286) -> ()  [unwired: 2 in, 2 out]
            n172 = property on="Test Ring" class="Ring (strict)"("Visible"=w286) -> ()  [unwired: 2 in, 2 out]
            n173 = Search and Replace String(input string=w287, search string="/Value  **", replace string="/Direction") -> (result string=w293:string)  [unwired: 5 in, 3 out]
            n174 = call <vilib>:"NT Read String.vi"("name"=w293) -> ("value"=w291:string)  [unwired: 8 in, 2 out]
            n175 = Equal?(x="Both directions", y=w291) -> (x = y?=w289:bool)
            n176 = property on="Rev/Fwd" class="Clust (strict)"("Visible"=w289) -> ()  [unwired: 2 in, 2 out]
            n177 = Not(x=w289) -> (.not. x?=w290:bool)
            n178 = property on="On/Off" class="Bool (strict)"("Visible"=w290, "Caption.Text"=w288) -> ()  [unwired: 2 in, 2 out]
          }
          frame "Compressor", "Digital Out" {
            w296 = FALSE ("Visible")
            # "Get direction and finish"
            n179 = property on="Test Ring" class="Ring (strict)"("Visible"=w296) -> ()  [unwired: 2 in, 2 out]
            n180 = property on="Motor" class="Clust (strict)"("Visible"=w296) -> ()  [unwired: 2 in, 2 out]
            n181 = property on="Test Slider" class="Slide (strict)"("Visible"=w296) -> ()  [unwired: 2 in, 2 out]
            n182 = property on="Rev/Fwd" class="Clust (strict)"("Visible"=FALSE) -> ()  [unwired: 2 in, 2 out]
            n183 = property on="On/Off" class="Bool (strict)"("Visible"=TRUE, "Caption.Text"=w297) -> ()  [unwired: 2 in, 2 out]
          }
          frame "Camera" {
            n184 = call <vilib>:"NT_Get Last Path Segment.vi"("String in"=w304) -> ("String out"=w305:string)  [unwired: 10 in]
            n185 = property on="On/Off" class="Bool (strict)"("Visible"=FALSE) -> ()  [unwired: 2 in, 2 out]
            n186 = case shown="\"White Balance  **\"" w305 {
              tunnel: w304 -> [w311 w320 w329 w338 w347 _ w353]
              tunnel: w303 -> [w309 w317 w326 w335 w344 _ _]
              frame "Size  **" {
                n187 = Index Array(array=w309) -> (element=w308:cluster{string[]})  [unwired: 1 in]
                n188 = call <vilib>:"NT Read String.vi"("name"=w311) -> ("value"=w310:string)  [unwired: 8 in, 2 out]
                n189 = property on="Test Slider" class="Slide (strict)"("Visible"=FALSE) -> ()  [unwired: 2 in, 2 out]
                n190 = property on="Test Ring" class="Ring (strict)"("Visible"=TRUE) -> ()  [unwired: 2 in, 2 out]
                n191 = Unbundle(w308) -> (w306:string[])
                n192 = Match First String(2:w306, 3:w310) -> (0:w307:i32)  [unwired: 1 out]
                n193 = property on="Test Ring" class="Ring (strict)"("Value"=w307, "Strings []"=w306) -> ()  [unwired: 2 in, 2 out]
              }
              frame "White Balance  **" {
                n194 = call <vilib>:"NT Read String.vi"("name"=w320) -> ("value"=w319:string)  [unwired: 8 in, 2 out]
                n195 = Index Array(array=w317, index=1) -> (element=w318:cluster{string[]})
                n196 = property on="Test Slider" class="Slide (strict)"("Visible"=FALSE) -> ()  [unwired: 2 in, 2 out]
                n197 = property on="Test Ring" class="Ring (strict)"("Visible"=TRUE) -> ()  [unwired: 2 in, 2 out]
                n198 = Unbundle(w318) -> (w315:string[])
                n199 = Match First String(2:w315, 3:w319) -> (0:w314:i32)  [unwired: 1 out]
                n200 = property on="Test Ring" class="Ring (strict)"("Value"=w314, "Strings []"=w315) -> ()  [unwired: 2 in, 2 out]
              }
              frame "Exposure  **" {
                n201 = call <vilib>:"NT Read String.vi"("name"=w329) -> ("value"=w328:string)  [unwired: 8 in, 2 out]
                n202 = Index Array(array=w326, index=2) -> (element=w327:cluster{string[]})
                n203 = property on="Test Slider" class="Slide (strict)"("Visible"=FALSE) -> ()  [unwired: 2 in, 2 out]
                n204 = property on="Test Ring" class="Ring (strict)"("Visible"=TRUE) -> ()  [unwired: 2 in, 2 out]
                n205 = Unbundle(w327) -> (w323:string[])
                n206 = Match First String(2:w323, 3:w328) -> (0:w324:i32)  [unwired: 1 out]
                n207 = property on="Test Ring" class="Ring (strict)"("Value"=w324, "Strings []"=w323) -> ()  [unwired: 2 in, 2 out]
              }
              frame "Exposure Priority  **" {
                n208 = call <vilib>:"NT Read String.vi"("name"=w338) -> ("value"=w337:string)  [unwired: 8 in, 2 out]
                n209 = Index Array(array=w335, index=3) -> (element=w336:cluster{string[]})
                n210 = property on="Test Slider" class="Slide (strict)"("Visible"=FALSE) -> ()  [unwired: 2 in, 2 out]
                n211 = property on="Test Ring" class="Ring (strict)"("Visible"=TRUE) -> ()  [unwired: 2 in, 2 out]
                n212 = Unbundle(w336) -> (w332:string[])
                n213 = Match First String(2:w332, 3:w337) -> (0:w333:i32)  [unwired: 1 out]
                n214 = property on="Test Ring" class="Ring (strict)"("Value"=w333, "Strings []"=w332) -> ()  [unwired: 2 in, 2 out]
              }
              frame "Color Enable  **" {
                n215 = call <vilib>:"NT Read String.vi"("name"=w347) -> ("value"=w346:string)  [unwired: 8 in, 2 out]
                n216 = Index Array(array=w344, index=4) -> (element=w345:cluster{string[]})
                n217 = property on="Test Slider" class="Slide (strict)"("Visible"=FALSE) -> ()  [unwired: 2 in, 2 out]
                n218 = property on="Test Ring" class="Ring (strict)"("Visible"=TRUE) -> ()  [unwired: 2 in, 2 out]
                n219 = Unbundle(w345) -> (w341:string[])
                n220 = Match First String(2:w341, 3:w346) -> (0:w342:i32)  [unwired: 1 out]
                n221 = property on="Test Ring" class="Ring (strict)"("Value"=w342, "Strings []"=w341) -> ()  [unwired: 2 in, 2 out]
              }
              frame Default {
                n222 = property on="Test Slider" class="Slide (strict)"("Visible"=FALSE) -> ()  [unwired: 2 in, 2 out]
                n223 = property on="Test Ring" class="Ring (strict)"("Visible"=FALSE) -> ()  [unwired: 2 in, 2 out]
              }
              frame "Brightness  **", "Color Level  **", "Compression  **", "FPS  **", "Sharpness  **" {
                n224 = call <vilib>:"NT Read Number.vi"("name"=w353) -> ("value"=w352:dbl)  [unwired: 8 in, 2 out]
                n225 = property on="Test Ring" class="Ring (strict)"("Visible"=FALSE) -> ()  [unwired: 2 in, 2 out]
                n226 = property on="Test Slider" class="Slide (strict)"("Visible"=TRUE, "Scale.Maximum"=100.0 ("Scale.Range:Maximum")) -> ()  [unwired: 2 in, 2 out]
                n227 = local write "Test Slider"(w352) -> ()
              }
            }
            n228 = property on="Motor" class="Clust (strict)"("Visible"=FALSE) -> ()  [unwired: 2 in, 2 out]
            n229 = property on="Rev/Fwd" class="Clust (strict)"("Visible"=FALSE) -> ()  [unwired: 2 in, 2 out]
          }
        }
      }
      event "Test Name": Mouse Enter {
        # "Populate the ring with the list of tests"
        n230 = event-data() -> ()  [unwired: 1 in, 1 out]
        n231 = call <vilib>:"NT Read String Array.vi"("name"="TestMode/TestList" ("Name")) -> ("value"=w360:string[])  [unwired: 8 in, 2 out]
        n232 = Build Array (concatenate)("Select the test to run...", w360) -> (w359:string[])
        n233 = property on="Test Name" class="Ring (strict)"("Strings []"=w359) -> ()  [unwired: 2 in, 2 out]
      }
      event "Test Name": Value Change {
        w361 = FALSE ("Visible")
        # "Tell the robot the test name to run"
        n234 = event-data() -> ("NewVal"=w365:u16)  [unwired: 1 in]
        n235 = property on="Test Name" class="Ring (strict)"() -> ("Strings []"=w366:string[])  [unwired: 2 in, 2 out]
        n236 = local write "Progress"(T6 {"Test Progress"=0, "Test Progress Text"=""} ("Progress")) -> ()
        n237 = Index Array(array=w366, index=w365) -> (element=w364:string)
        n238 = property on="Progress" class="Clust (strict)"("Visible"=TRUE) -> ()  [unwired: 2 in, 2 out]
        n239 = property on="Test Ring" class="Ring (strict)"("Visible"=w361) -> ()  [unwired: 2 in, 2 out]
        n240 = property on="Motor" class="Clust (strict)"("Visible"=w361) -> ()  [unwired: 2 in, 2 out]
        n241 = property on="Test Slider" class="Slide (strict)"("Visible"=w361) -> ()  [unwired: 2 in, 2 out]
        n242 = property on="On/Off" class="Bool (strict)"("Visible"=w361) -> ()  [unwired: 2 in, 2 out]
        n243 = property on="Rev/Fwd" class="Clust (strict)"("Visible"=w361) -> ()  [unwired: 2 in, 2 out]
        n244 = call <vilib>:"NT Write String.vi"("value"=w364, "name"="TestMode/TestName" ("Name")) -> ()  [unwired: 9 in, 1 out]
      }
      event "Select Auto": Mouse Enter {
        # "Populate the combo box with the list of autonomous options"
        n245 = event-data() -> ()  [unwired: 1 in, 1 out]
        n246 = call <vilib>:"NT Read String Array.vi"("name"="Auto List" ("Name")) -> ("value"=w368:string[])  [unwired: 8 in, 2 out]
        n247 = property on="Select Auto" class="CmbBox"("Strings[]"=w368) -> ()  [unwired: 2 in, 2 out]
      }
      event "Select Auto": Value Change {
        # "User modified the Auto Selection. Write to NT variable so robot knows."
        n248 = event-data() -> ("NewVal"=w370:string)  [unwired: 1 in]
        n249 = call <vilib>:"NT Write String.vi"("value"=w370, "name"="Auto Selector" ("Name")) -> ()  [unwired: 9 in, 1 out]
      }
      event "CheckList": Double Click {
        # "Shift clears all"
        # "Update symbols on the listbox"
        n250 = event-data() -> ("PlatMods.Shift"=w372:bool, "Row"=w374:i32)  [unwired: 1 in]
        n251 = case shown="True" w372 {
          tunnel: w374 -> [w378 _]
          tunnel: 1 -> [w377 _]
          frame False {
            n252 = property on="CheckList" class="LstBox (strict)"() -> ("Item Symbols"=w376:i32[])  [unwired: 2 in, 2 out]
            n253 = Replace Array Subset(array=w376, new element=w377, index=w378) -> (w375:i32[])
            n254 = property on="CheckList" class="LstBox (strict)"("Item Symbols"=w375) -> ()  [unwired: 2 in, 2 out]
          }
          frame True {
            w379 = 0 ("Top Row")
            n255 = property on="CheckList" class="LstBox (strict)"() -> ("Number of Rows"=w381:u32)  [unwired: 2 in, 2 out]
            n256 = Initialize Array(0, w381) -> (w380:i32[])
            n257 = property on="CheckList" class="LstBox (strict)"("Top Row"=w379, "Value"=w379, "Item Symbols"=w380) -> ()  [unwired: 2 in, 2 out]
          }
        }
      }
      event "CheckList": Key Down {
        # "Update symbols on the listbox\nLeft and right keys check and uncheck"
        n258 = event-data() -> ("VKey"=w384:T22)  [unwired: 1 in]
        n259 = case shown="\"Left\", \"Right\"" w384 {
          selector: w384 -> [w389 _]
          tunnel: eventvkey."Left" ("VKey") -> [w387 _]
          frame "Left", "Right" {
            n260 = Equal?(x=w387, y=w389) -> (x = y?=w388:bool)
            n261 = Select(t=0, s=w388, f=1) -> (s? t:f=w390:i32)
            n262 = property on="CheckList" class="LstBox (strict)"() -> ("Item Symbols"=w393:i32[])  [unwired: 2 in, 2 out]
            n263 = Replace Array Subset(array=w393, new element=w390, index="CheckList") -> (w392:i32[])
            n264 = property on="CheckList" class="LstBox (strict)"("Item Symbols"=w392) -> ()  [unwired: 2 in, 2 out]
          }
          frame Default {
          }
        }
      }
      event "Motor.Enable": Value Change {
        # "When the test mode otor enable helper is set, update that\ntree row item's value"
        n265 = event-data() -> ("NewVal"=w398:bool)  [unwired: 1 in]
        n266 = Unbundle("Motor") -> ("Value"=w397:dbl)  [unwired: 1 out]
        n267 = Select(t=w397, s=w398, f=0.0) -> (s? t:f=w395:dbl)
        n268 = call <vilib>:"NT Write Number.vi"("value"=w395, "name"=w394) -> ()  [unwired: 9 in, 1 out]
      }
      event "Test Slider": Value Change {
        # "When the test mode slider helper is set, update that\ntree row item's value"
        n269 = event-data() -> ("NewVal"=w400:dbl)  [unwired: 1 in]
        n270 = call <vilib>:"NT Write Number.vi"("value"=w400, "name"=w401) -> ()  [unwired: 9 in, 1 out]
      }
      event "On/Off": Value Change {
        # "When the test mode on/off helper value is set, update that\ntree row item's value"
        n271 = event-data() -> ("NewVal"=w404:bool)  [unwired: 1 in]
        n272 = Boolean To (0,1)(Boolean=w404) -> (0, 1=w403:i16)
        n273 = call <vilib>:"NT Write Number.vi"("value"=w403, "name"=w402) -> ()  [unwired: 9 in, 1 out]
      }
      event "Rev/Fwd": Value Change {
        # "When the test mode helper value for relays is set, update that\ntree row item's value"
        n274 = event-data() -> ("NewVal.Forward"=w411:bool, "NewVal.Reverse"=w410:bool)  [unwired: 1 in]
        n275 = Boolean To (0,1)(Boolean=w411) -> (0, 1=w407:i16)
        n276 = Boolean To (0,1)(Boolean=w410) -> (0, 1=w409:i16)
        n277 = Negate(x=w409) -> (-x=w408:i16)
        n278 = Add(x=w407, y=w408) -> (x+y=w406:i16)
        n279 = call <vilib>:"NT Write Number.vi"("value"=w406, "name"=w405) -> ()  [unwired: 9 in, 1 out]
      }
      event "Test Ring": Value Change {
        # "When a test mode helper value is selected from the ring,\nset the tree item's variable to the string value"
        n280 = event-data() -> ("NewVal"=w414:u16)  [unwired: 1 in]
        n281 = property on="Test Ring" class="Ring (strict)"() -> ("Strings []"=w415:string[])  [unwired: 2 in, 2 out]
        n282 = Index Array(array=w415, index=w414) -> (element=w413:string)
        n283 = call <vilib>:"NT Write String.vi"("value"=w413, "name"=w412) -> ()  [unwired: 9 in, 1 out]
      }
      event "Rec Mode": Value Change {
        # "Update globals for recording mode and path to read log from.\nClear when logging and let NetworkTables set path for vision to\nuse."
        n284 = event-data() -> ("NewVal"=w424:enum32{"Stop", "Record", "Playback"})  [unwired: 1 in]
        n285 = global write "WPI_DashboardLogging Global.vi" "Recording"(w424) -> ()
        n286 = global write "WPI_DashboardLogging Global.vi" "Logging Filename"(path "") -> ()
        n287 = case shown="\"Playback\"" w424 {
          tunnel: w423 -> [_ w426 w434]
          tunnel: [_ _ w433] -> w421
          tunnel: [_ _ w432] -> _
          tunnel: w419 -> [_ _ w430]
          tunnel: cluster{i32, i32} {-250, 170} -> [_ _ w429]
          tunnel: [_ _ T23 {"Image Size"=TRUE, "Image Type"=TRUE, "Pixel Value"=TRUE, "ROI Information"=TRUE, "Zoom Factor"=FALSE} ("Image Information Shown:All Elements")] -> w416
          tunnel: [_ _ TRUE ("Zoom Factor")] -> w417
          frame Default {
          }
          frame "Stop", "Record" {
            # "Place Window too"
            n288 = invoke class="VI" method="FP.Close"(reference=w426) -> (reference out=w425:refnum<vi>)  [unwired: 2 in, 2 out]
            n289 = invoke class="VI" method="Abort VI"(reference=w425) -> ()  [unwired: 2 in, 3 out]
          }
          frame "Playback" {
            n290 = call "Open Playback Panel.vi"("Offset"=w429, "DB VI Ref"=w430, "Playback in"=w434) -> ("Playback out"=w431:refnum<vi>)  [unwired: 8 in]
            n291 = register-events(w431) -> (reference out=w433:refnum<event-registration>, error out=w432:errorcluster)  [unwired: 2 in]
          }
        }
        n292 = call <vilib>:"WPI_DashboardNT Log FieldName Cache.vi"("Operation"=enum16{"Lookup/Add", "Index", "Clear"}."Clear") -> ()  [unwired: 8 in, 3 out]
        n293 = property on="Camera Image" class="ImageControl"("Image Information Shown"=w416, "Image Information Visible"=w417) -> ()  [unwired: 2 in, 2 out]
        n294 = property on="Camera Image Right" class="ImageControl"("Image Information Shown"=w416, "Image Information Visible"=w417) -> ()  [unwired: 2 in, 2 out]
      }
      event Panel Close {
        w435 = enum32{"Stop", "Record", "Playback"}."Stop" ("Rec Mode")
        # "Playback window has been closed, abort"
        n295 = event-data() -> ()  [unwired: 1 in, 4 out]
        n296 = local write "Rec Mode"(w435) -> ()
        n297 = global write "WPI_DashboardLogging Global.vi" "Recording"(w435) -> ()
      }
      event Panel Close {
        # "Abort playback window and ourself"
        n298 = event-data() -> ()  [unwired: 1 in, 4 out]
        n299 = invoke class="VI" method="FP.Close"(reference=w438) -> (reference out=w437:refnum<vi>)  [unwired: 2 in, 2 out]
        n300 = invoke class="VI" method="Abort VI"(reference=w437) -> (error out=w436:errorcluster)  [unwired: 2 in, 2 out]
        n301 = invoke class="VI" method="Abort VI"(error in=w436) -> ()  [unwired: 2 in, 3 out]
      }
      event "Tree": Double Click {
        n302 = event-data() -> ("PlatMods"=w444:T25, "Tag"=w441:string)  [unwired: 1 in]
        n303 = Unbundle(w444) -> ("Shift"=w443:bool)  [unwired: 4 out]
        n304 = Not(x=w443) -> (.not. x?=w442:bool)
        n305 = String Subset(string=w441, length (rest)=1 ("length (rest)")) -> (substring=w440:string)  [unwired: 1 in]
        n306 = case shown="\"/\"" w440 {
          tunnel: w441 -> [_ w446]
          tunnel: w442 -> [_ w445]
          frame Default {
          }
          frame "/" {
            n307 = call <vilib>:"NT Update Persistence.vi"("Persistence"=w445, "Name"=w446) -> ()  [unwired: 9 in, 1 out]
          }
        }
      }
    }
  }
